vi "TCP - Read LineFeed Terminated String.vi"(8 "error in":errorcluster, 11 "TCP Network Connection in":refnum<k5>) -> (0 "error out":errorcluster, 2 "Received Text":string, 3 "TCP Network Connection out":refnum<k5>)   [LabVIEW 2020]
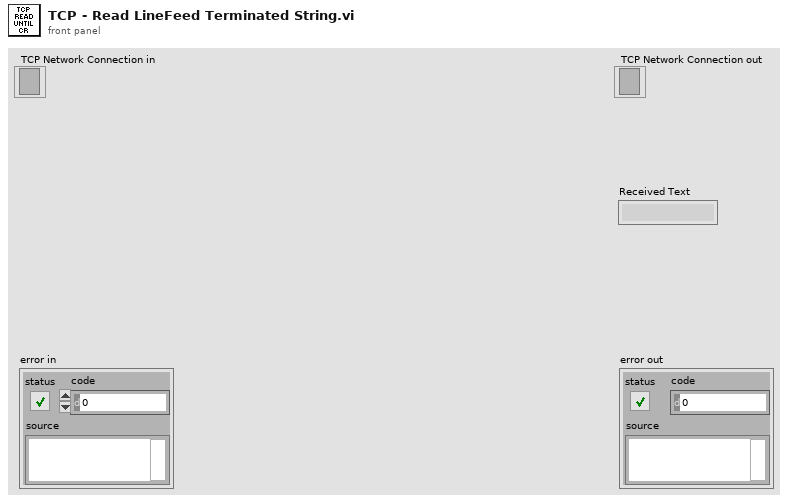
[diagram p1: front panel]
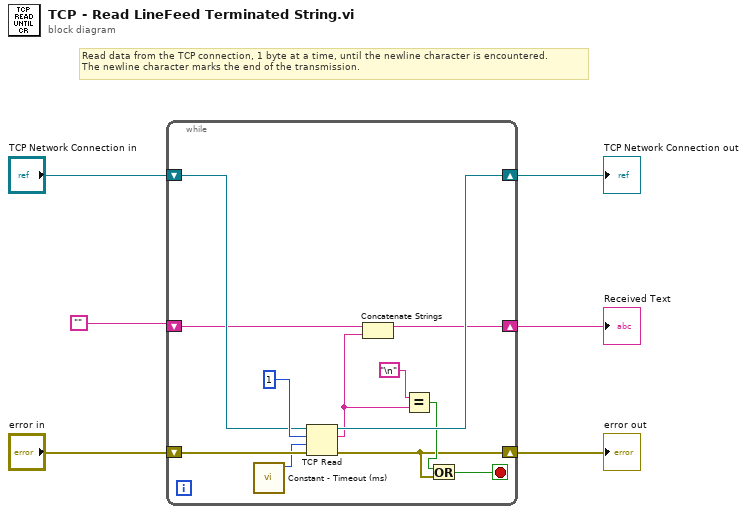
[diagram p0: block diagram]
diagram:
  # "Read data from the TCP connection, 1 byte at a time, until the newline character is encountered.\nThe newline character marks the end of the transmission."
  n1 = while {
    shift-right: [w9] -> w5
    shift-left: "error in" -> [w18]
    shift-right: [w15] -> w3
    shift-left: "TCP Network Connection in" -> [w16]
    shift-right: [w12] -> w1
    shift-left: "" -> [w14]
    stop <- w8 stop-if-true
    n2 = call "Constant - Timeout (ms).vi"() -> ("timeout (ms)"=w11:i32)  [unwired: 11 in]
    n3 = TCP Read(connection ID=w16, bytes to read=1, error in (no error)=w18, 9:w11) -> (connection ID out=w15:refnum<k5>, data out=w13:string, error out=w9:errorcluster)  [unwired: 1 in]
    n4 = Concatenate Strings(w14, w13) -> (w12:string)
    n5 = Equal?(x="\n", y=w13) -> (x = y?=w10:bool)
    n6 = Or(x=w10, y=w9) -> (x .or. y?=w8:bool)
  }
  "TCP Network Connection out" <- w3
  "error out" <- w5
  "Received Text" <- w1
